vi "Scan1.vi"() -> ()   [LabVIEW 2022 SP3]
uses:
  <vilib>/userdefined/High Color/IMAQdx.ctl
  <vilib>/Utility/file.llb/Write To Spreadsheet File (DBL).vi
  <vilib>/vision/driver/NI_Vision_Acquisition_Software.lvlib
  <resource>/objmgr/IMAQImage.rc
panel:
  in  "ExitSendCmd":bool
  out "Current File":path
  in  "Root File Name":string="Sample"
  in  "Display as wavelngth?":bool=TRUE
  in  "ActiveFlyCapControl":refnum<k7>(container)
  out "X axis":dbl[](array[numeric])
  in  "Tab Control":enum32{"Scan", "Motors"}(tab)
  in  "Save Option":bool=TRUE
  out "Remaining Minutes":i32
  out "Progress Bar":dbl(slide) scale=0.0..1.0
  in  "Sample #":u16
  out "Cross Plane Length (mm)":sgl=128.0 format="%.3f"
  out "Scan Plane Length (mm)":sgl=128.0 format="%.3f"
  in  "Distance between\nscan lines (mm)":sgl=1.0 min=0.06 max=1000 step=0.06
  in  "Distance between\nplanes (mm)":sgl=1.0 min=0.06 max=1000 step=0.06
  in  "number of planes":u16=1660
  in  "lines per plane":u16=1660 min=1
  out "current plane":u16
  out "current line":u16
  in  "Abort":bool
  in  "start scan":bool
  out "Image":T1(plugin-control)
  out "Spectra":cluster{"X":dbl[], "Spectral Amplitude":dbl[]}(graph)
  in  "Save Folder":path=path "D:/Scan Test"
  in  "Average#":i32=1 min=1
  in  "Exposure (*2.375 ms)":u16=2 format="%.3f"
  in  "Plane Axis":refnum<k7>(container)
  in  "Line axis":refnum<k7>(container)
  in  "Home Seq":bool
  in  "Go Home":bool
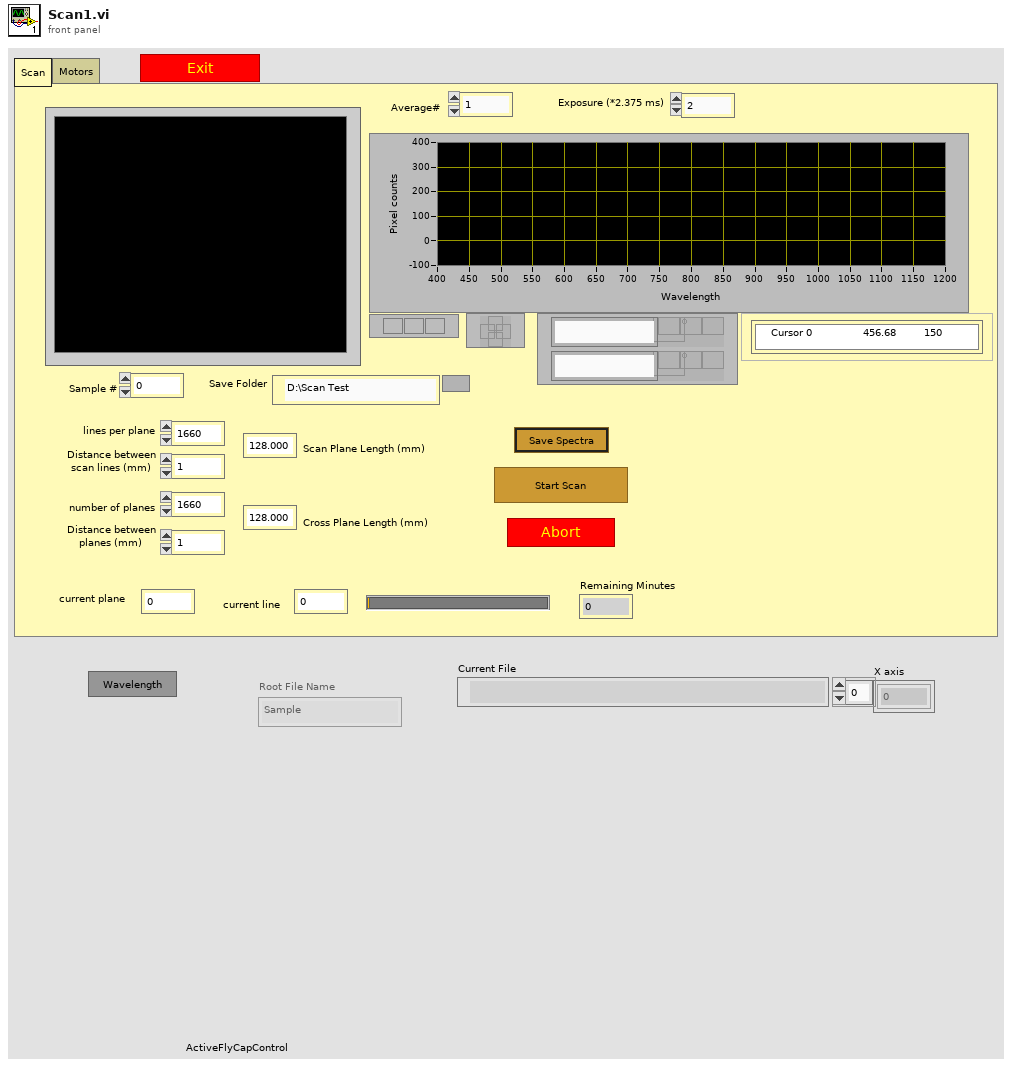
[diagram p1: front panel]
types:
  T1 = typedef "IMAQ Image.ctl" = refnum<image>
  T2 = typedef "IMAQdx.ctl" = refnum<k21>
  T3 = typedef "Image Type" = u32
  T4 = cluster{"X axis":dbl[], "Spectral Amplitude":dbl[]}
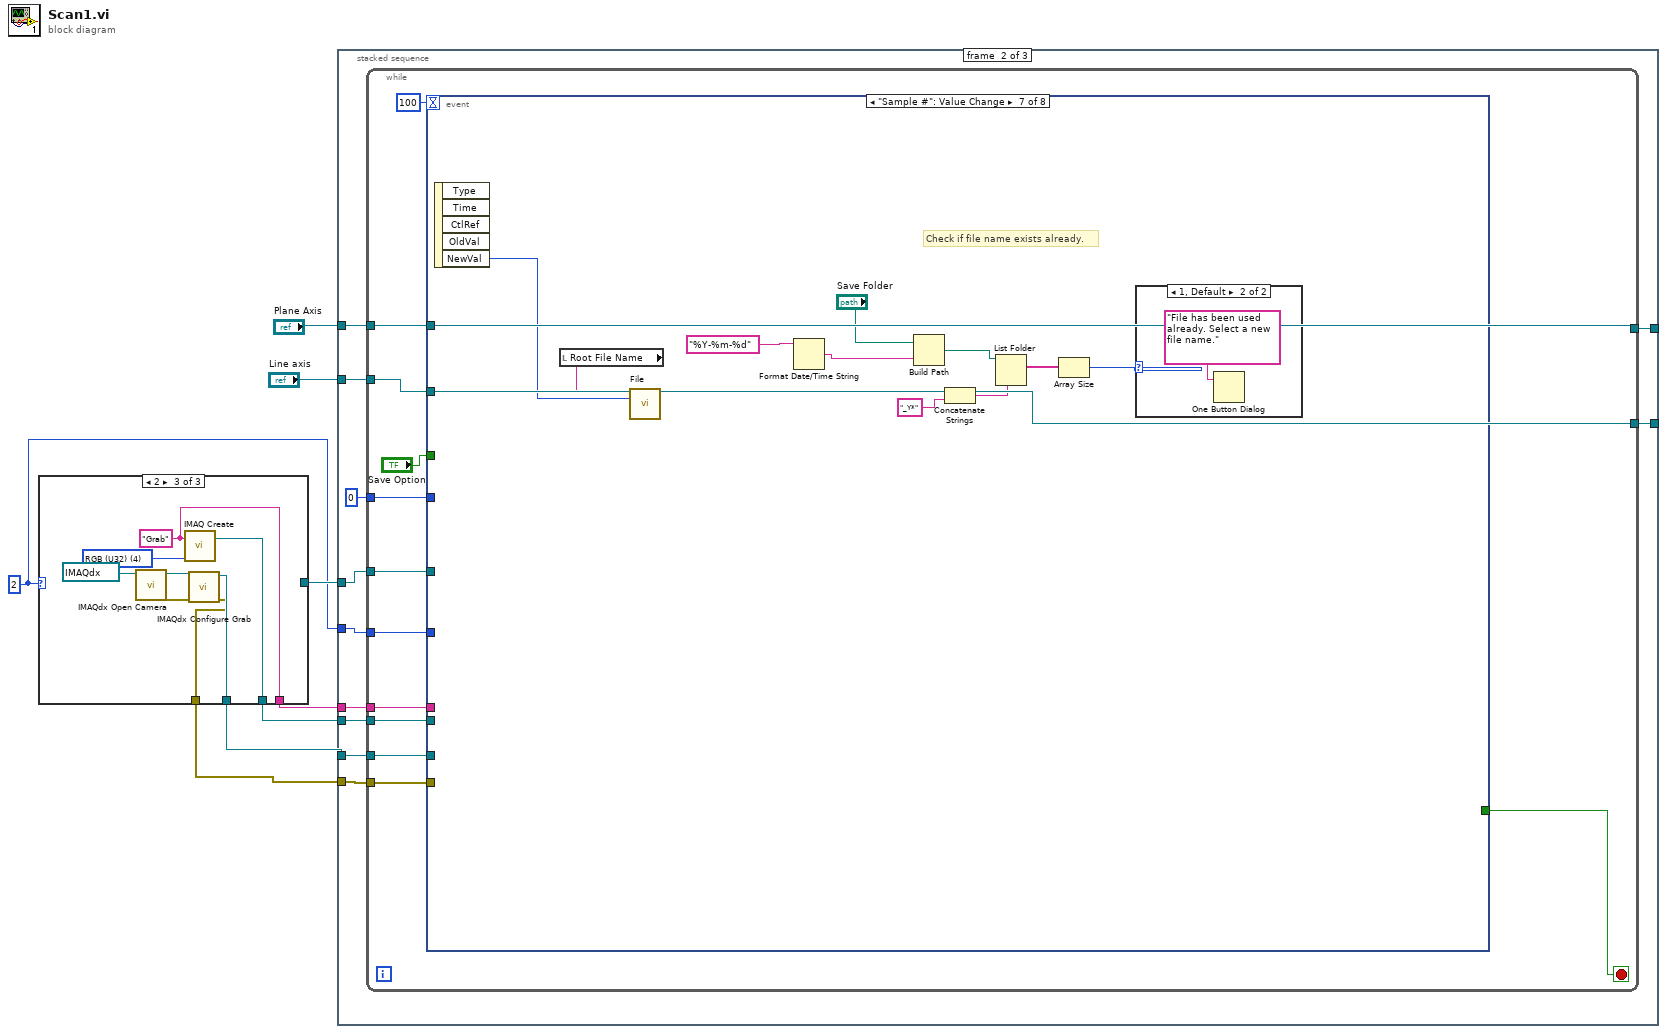
[diagram p0: block diagram]
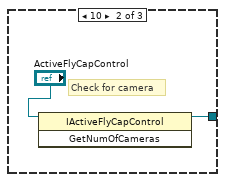
[diagram p3: hidden frame]
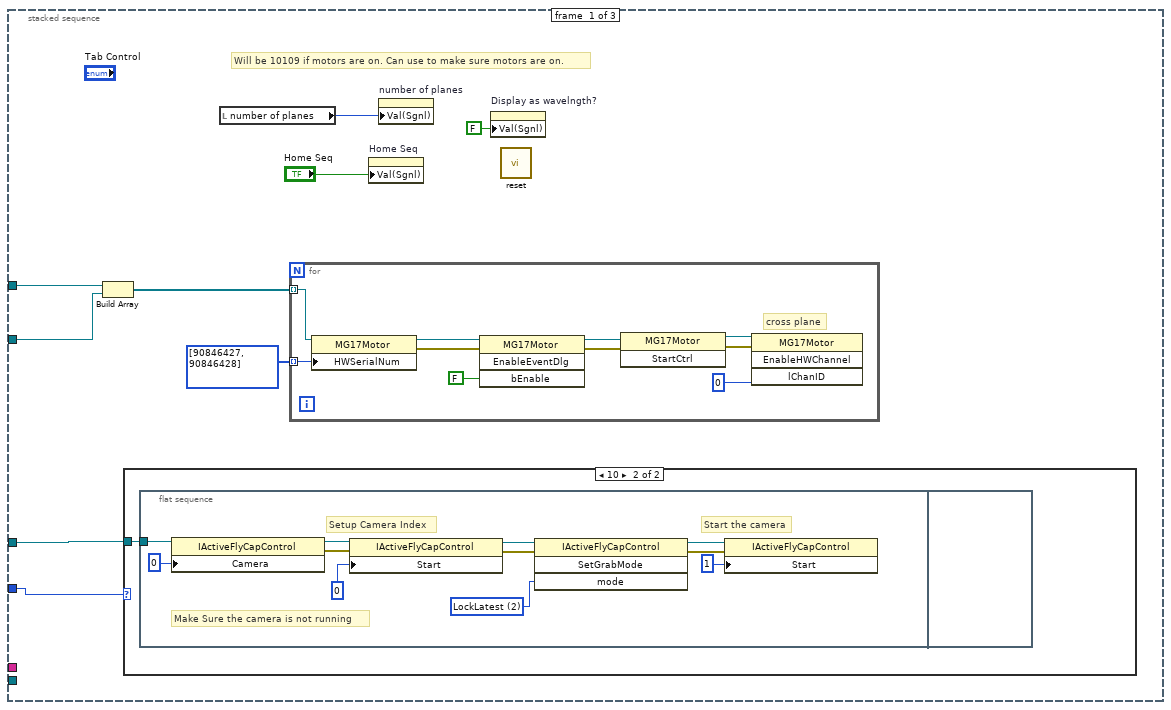
[diagram p4: hidden frame]
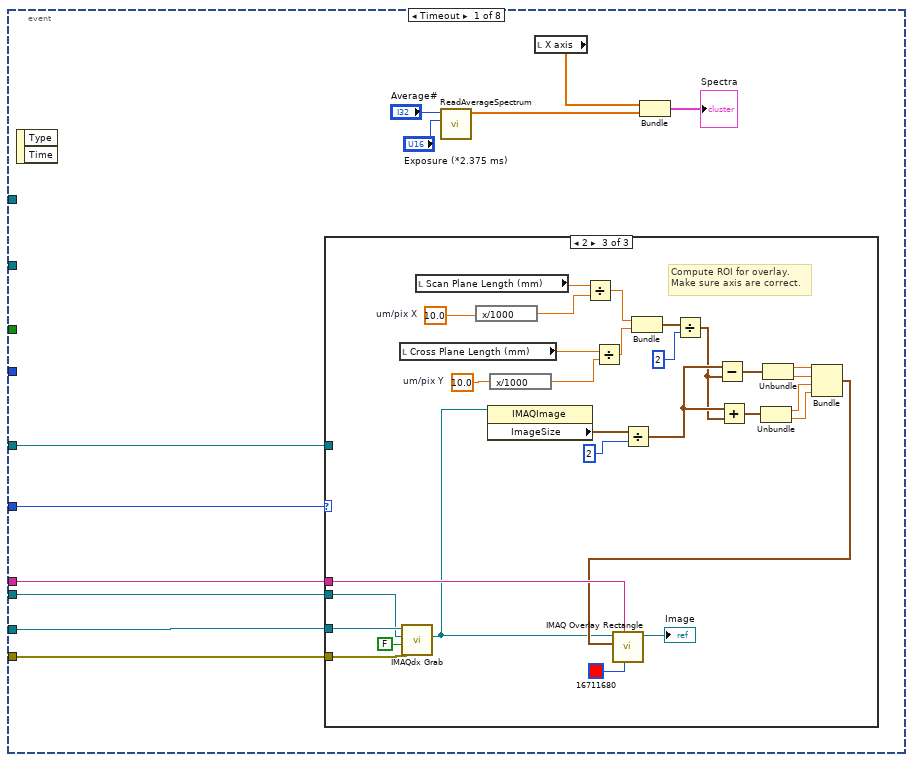
[diagram p6: hidden frame]
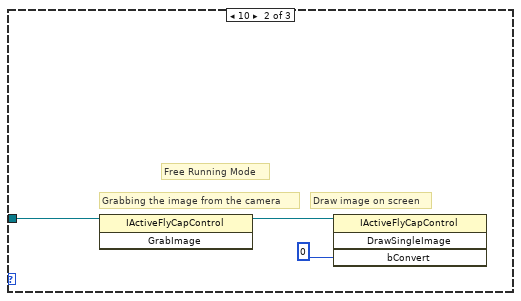
[diagram p8: hidden frame]
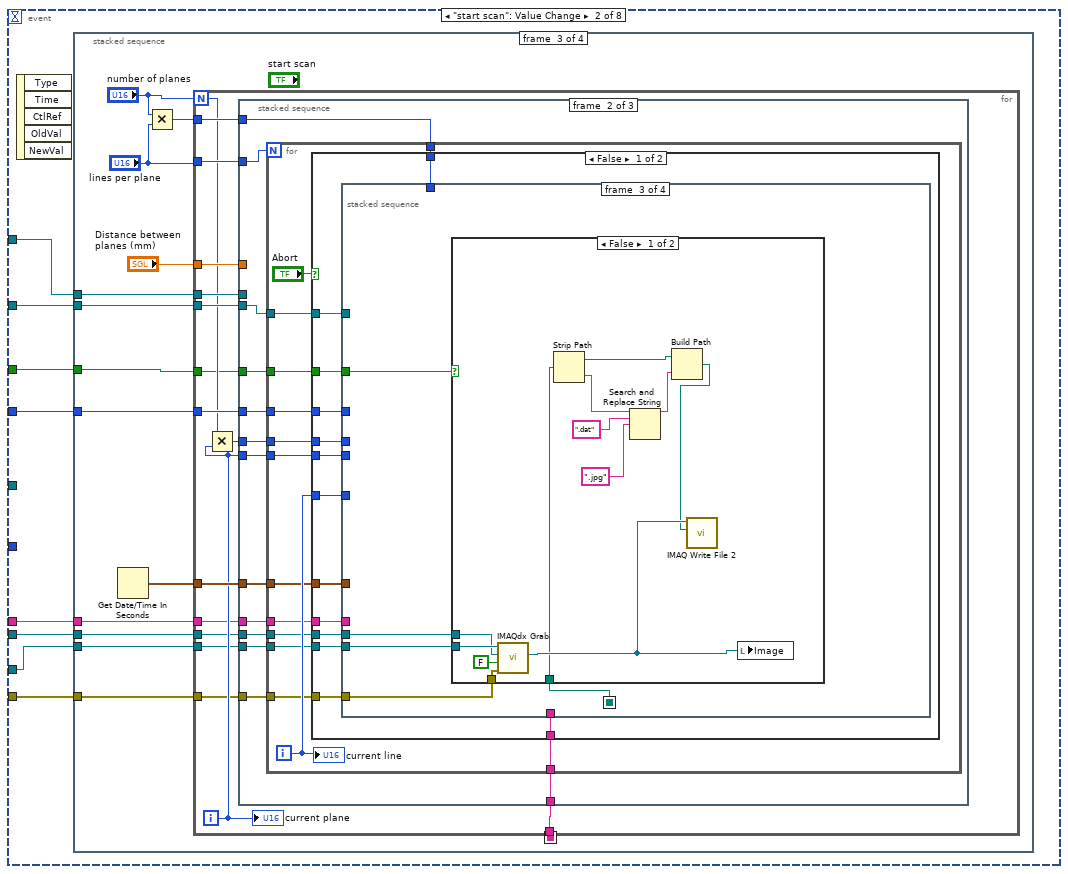
[diagram p9: hidden frame]
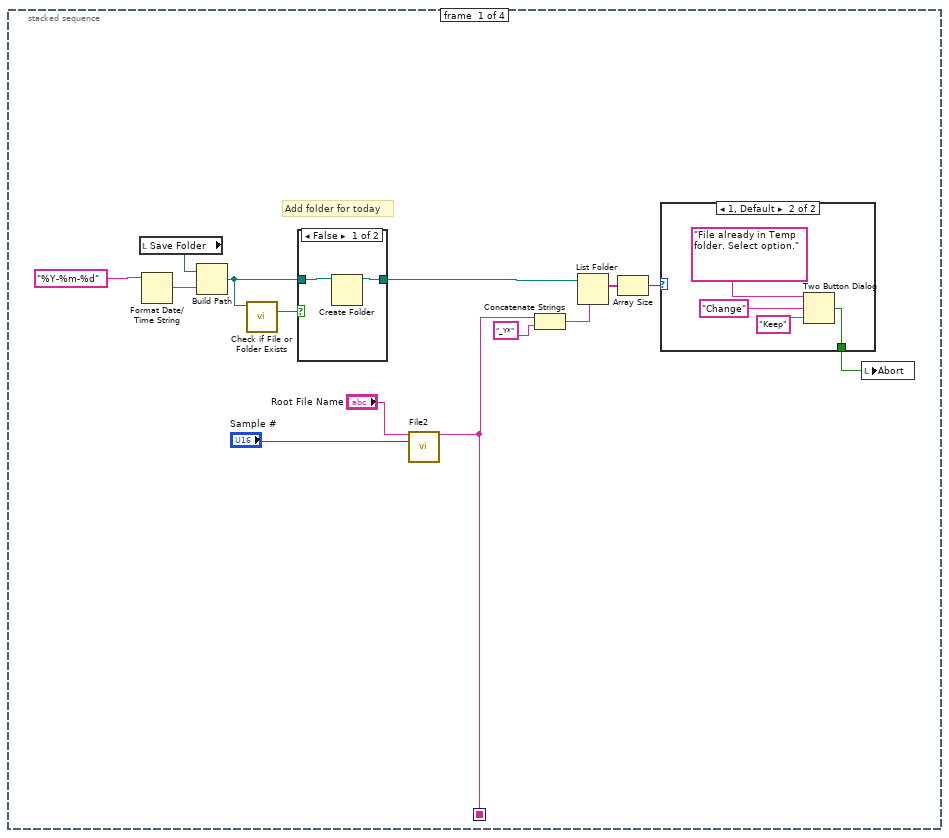
[diagram p10: hidden frame]
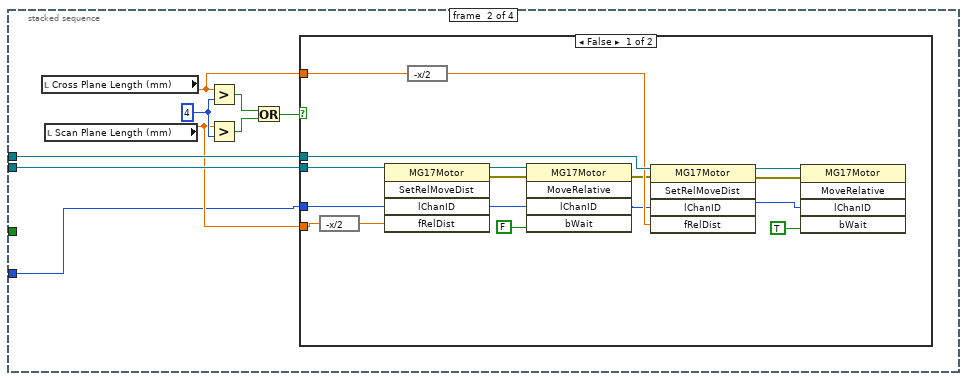
[diagram p13: hidden frame]
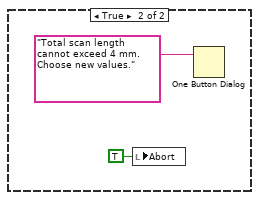
[diagram p14: hidden frame]
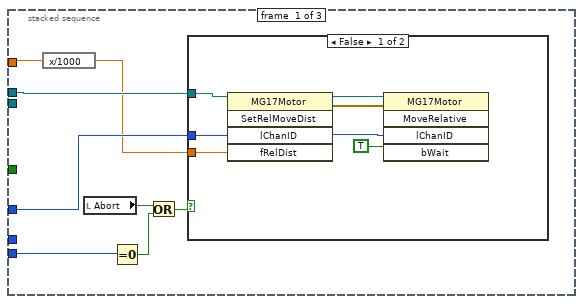
[diagram p15: hidden frame]
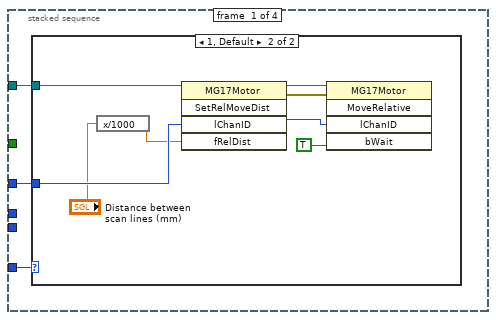
[diagram p17: hidden frame]
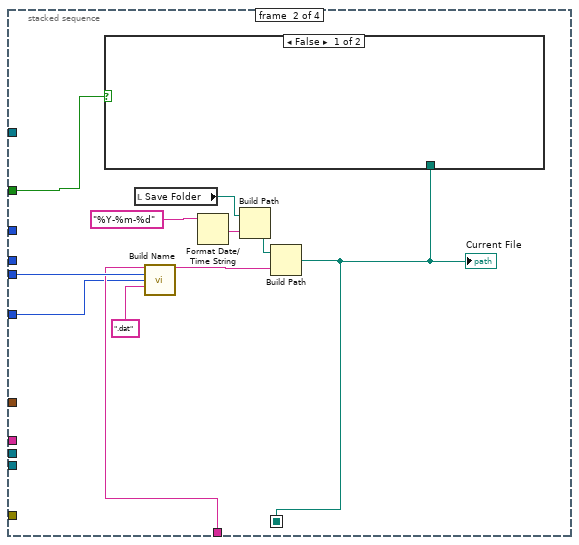
[diagram p19: hidden frame]
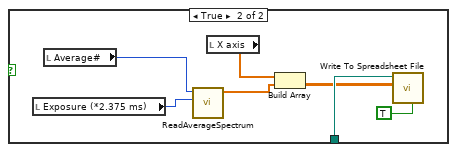
[diagram p20: hidden frame]
diagram:
  w1 = 2 ("bConvert")
  n1 = case shown="2" w1 {
    tunnel: [_ w10 _] -> w6
    tunnel: [_ _ w14] -> w5
    tunnel: [_ _ w13] -> w4
    tunnel: [_ _ w12] -> w3
    tunnel: [_ _ w11] -> w2
    frame 0, Default {
    }
    frame 10 {
      # "Check for camera"
      n2 = invoke class="IActiveFlyCapControl" method="GetNumOfCameras"(reference="ActiveFlyCapControl") -> (reference out=w10:refnum<k7>)  [unwired: 2 in, 2 out]
    }
    frame 2 {
      w15 = T3 4 items=["Grayscale (U8)", "Grayscale (I16)", "Grayscale (SGL)", "Complex (CSG)", "RGB (U32)", "HSL (U32)", "RGB (U64)", "Grayscale (U16)"] ("Image Type")
      w14 = "Grab" ("Image Name")
      n3 = call <vilib>:"IMAQdx Open Camera.vi"("Session In"=T2 "cam1") -> ("error out"=w17:errorcluster, "Session Out"=w18:T2)  [unwired: 2 in, 7 out]
      n4 = call "IMAQ Create"("Image Name"=w14, "Image Type"=w15) -> ("New Image"=w13:T1)  [unwired: 2 in, 2 out]
      n5 = call <vilib>:"IMAQdx Configure Grab.vi"("error in"=w17, "Session In"=w18) -> ("error out"=w11:errorcluster, "Session Out"=w12:T2)  [unwired: 1 in, 7 out]
    }
  }
  n6 = stacked-sequence {
    tunnel: [_ w59 _] -> _
    tunnel: [_ w58 _] -> _
    tunnel: w6 -> [w22 w57 w432]
    tunnel: "Plane Axis" -> [w20 w56 w431]
    tunnel: "Line axis" -> [w21 w55 w430]
    tunnel: w3 -> [_ w54 w428]
    tunnel: w4 -> [_ w53 w429]
    tunnel: w2 -> [_ w51 w427]
    tunnel: w5 -> [_ w52 _]
    tunnel: w1 -> [w19 w50 w426]
    frame #0 {
      # "Will be 10109 if motors are on. Can use to make sure motors are on."
      n7 = Build Array(w20, w21) -> (w23:refnum<k7>[])
      n8 = case shown="10" w19 {
        tunnel: w22 -> [_ w28]
        frame 0, Default {
        }
        frame 10 {
          n9 = flat-sequence {
            tunnel: w28 -> [w29]
            frame #0 {
              w32 = 2 items=["FreeRunning", "LockNext", "LockLatest"] ("mode")
              # "Make Sure the camera is not running"
              # "Setup Camera Index"
              # "Start the camera"
              n10 = property class="IActiveFlyCapControl"(reference=w29, "Camera"=0 ("Start")) -> (reference out=w35:refnum<k7>, error out=w37:errorcluster)  [unwired: 1 in]
              n11 = property class="IActiveFlyCapControl"(reference=w35, error in=w37, "Start"=0 ("Camera")) -> (reference out=w33:refnum<k7>, error out=w34:errorcluster)
              n12 = invoke class="IActiveFlyCapControl" method="SetGrabMode"(reference=w33, error in=w34, "mode"=w32) -> (reference out=w36:refnum<k7>, error out=w38:errorcluster)  [unwired: 1 in, 2 out]
              n13 = property class="IActiveFlyCapControl"(reference=w36, error in=w38, "Start"=1) -> ()  [unwired: 2 out]
            }
            frame #1 {
            }
          }
        }
      }
      n14 = local read "number of planes"() -> (w26:u16)
      n15 = for {
        tunnel: i32[] [90846427, 90846428] -> [w41] mode=indexing
        tunnel: w23 -> [w42] mode=indexing
        # "cross plane"
        n16 = property class="MG17Motor"(reference=w42, "HWSerialNum"=w41) -> (reference out=w40:refnum<k7>, error out=w45:errorcluster)  [unwired: 1 in]
        n17 = invoke class="MG17Motor" method="EnableEventDlg"(reference=w40, error in=w45, "bEnable"=FALSE ("pbCommsOK")) -> (reference out=w44:refnum<k7>, error out=w43:errorcluster)  [unwired: 1 in, 2 out]
        n18 = invoke class="MG17Motor" method="StartCtrl"(reference=w44, error in=w43) -> (reference out=w49:refnum<k7>, error out=w48:errorcluster)  [unwired: 1 in, 1 out]
        n19 = invoke class="MG17Motor" method="EnableHWChannel"(reference=w49, error in=w48, "lChanID"=0) -> ()  [unwired: 1 in, 4 out]
      }
      n20 = property on="Home Seq" class="Bool (strict)"("Val(Sgnl)"="Home Seq") -> ()  [unwired: 2 in, 2 out]
      n21 = property on="number of planes" class="DigNum (strict)"("Val(Sgnl)"=w26) -> ()  [unwired: 2 in, 2 out]
      n22 = property on="Display as wavelngth?" class="Bool (strict)"("Val(Sgnl)"=FALSE ("Value (Signaling)")) -> ()  [unwired: 2 in, 2 out]
      n23 = call "reset.vi"() -> ()  [unwired: 1 in]
    }
    frame #1 {
      n24 = while {
        tunnel: w55 -> [w69]
        tunnel: w56 -> [w70]
        tunnel: 0 ("lChanID") -> [w71]
        tunnel: [w69] -> w59
        tunnel: [w70] -> w58
        tunnel: w57 -> [w67]
        tunnel: w54 -> [w65]
        tunnel: w53 -> [w66]
        tunnel: w52 -> [w64]
        tunnel: w51 -> [w63]
        tunnel: w50 -> [w62]
        stop <- w72 stop-if-true
        n25 = event shown="[6] \"Sample #\": Value Change" {
          selector: _ -> [_ _ _ _ _ _ _ _]
          dyn-events: _ -> [_ _ _ _ _ _ _ _]
          timeout: 100 -> [_ _ _ _ _ _ _ _]
          tunnel: w69 -> [_ w121 w338 _ w371 _ _ _]
          tunnel: w70 -> [_ w123 w337 _ w372 _ _ _]
          tunnel: [_ _ _ "ExitSendCmd" _ _ _ _] -> w72
          tunnel: w71 -> [_ w122 w333 _ w368 _ _ _]
          tunnel: w67 -> [w83 _ _ _ _ _ _ _]
          tunnel: w66 -> [w76 w118 _ _ _ _ _ _]
          tunnel: w65 -> [w77 w120 _ _ _ _ _ _]
          tunnel: w64 -> [w75 w117 _ _ _ _ _ _]
          tunnel: w63 -> [w74 w119 _ _ _ _ _ _]
          tunnel: w62 -> [w73 _ _ _ _ _ _ _]
          tunnel: "Save Option" -> [_ w116 _ _ _ _ _ _]
          event Timeout {
            n26 = event-data() -> ()  [unwired: 1 in, 2 out]
            n27 = case shown="2" w73 {
              tunnel: w83 -> [_ w85 _]
              tunnel: w77 -> [_ _ w112]
              tunnel: w76 -> [_ _ w109]
              tunnel: w75 -> [_ _ w114]
              tunnel: w74 -> [_ _ w110]
              frame 0, Default {
              }
              frame 10 {
                # "Draw image on screen"
                # "Grabbing the image from the camera"
                # "Free Running Mode"
                n28 = invoke class="IActiveFlyCapControl" method="GrabImage"(reference=w85) -> (reference out=w84:refnum<k7>)  [unwired: 2 in, 2 out]
                n29 = invoke class="IActiveFlyCapControl" method="DrawSingleImage"(reference=w84, "bConvert"=0) -> ()  [unwired: 2 in, 4 out]
              }
              frame 2 {
                w104 = 10.0  # um/pix Y
                w105 = 10.0  # um/pix X
                # "Compute ROI for overlay.\nMake sure axis are correct."
                n30 = local read "Cross Plane Length (mm)"() -> (w88:sgl)
                n31 = call <vilib>:"IMAQdx Grab.vi"("error in"=w110, "Wait for Next Buffer? (Yes)"=FALSE, "Image In"=w109, "Session In"=w112) -> ("Image Out"=w89:T1)  [unwired: 7 out]
                n32 = local read "Scan Plane Length (mm)"() -> (w106:sgl)
                n33 = expression code="x/1000"(w105) -> (w103:dbl)
                n34 = property class="IMAQImage"(reference=w89) -> ("ImageSize"=w108:cluster{"x":i32, "y":i32})  [unwired: 1 in, 2 out]
                n35 = expression code="x/1000"(w104) -> (w87:dbl)
                n36 = Divide(x=w106, y=w103) -> (x/y=w102:dbl)
                n37 = Divide(x=w88, y=w87) -> (x/y=w101:dbl)
                n38 = Divide(x=w108, y=2) -> (x/y=w98:cluster{"x":dbl, "y":dbl})
                n39 = Bundle(w102, w101) -> (w100:cluster{dbl, dbl})  [unwired: 1 in]
                n40 = Divide(x=w100, y=2) -> (x/y=w97:cluster{dbl, dbl})
                n41 = Subtract(x=w98, y=w97) -> (x-y=w96:cluster{dbl, dbl})
                n42 = Add(x=w98, y=w97) -> (x+y=w95:cluster{dbl, dbl})
                n43 = Unbundle(w95) -> (w92:dbl, w91:dbl)
                n44 = Unbundle(w96) -> (w94:dbl, w93:dbl)
                n45 = Bundle(w94, w93, w92, w91) -> (w90:cluster{dbl, dbl, dbl, dbl})  [unwired: 1 in]
                n46 = call "IMAQ Overlay Rectangle"("Color"=u32 16711680, "Group"=w114, "Rectangle"=w90, "Image"=w89) -> ("Image Out"=→"Image":T1)  [unwired: 6 in, 1 out]
              }
            }
            n47 = call "ReadAverageSpectrum.vi"("Exposure (*2.375 ms)"="Exposure (*2.375 ms)", "Average#"="Average#") -> ("Spectral Amplitude"=w78:dbl[])  [unwired: 9 in]
            n48 = local read "X axis"() -> (w82:dbl[])
            n49 = Bundle("X axis"=w82, "Spectral Amplitude"=w78) -> (→"Spectra":T4)  [unwired: 1 in]
          }
          event "start scan": Value Change {
            n50 = event-data() -> ()  [unwired: 1 in, 5 out]
            n51 = stacked-sequence {
              seq-local: [w129 _ _ _] -> [_ _ w182 _]
              tunnel: w123 -> [_ w149 w186 _]
              tunnel: w121 -> [_ w150 w184 _]
              tunnel: w122 -> [_ w145 w183 _]
              tunnel: w120 -> [_ _ w177 _]
              tunnel: w119 -> [_ _ w176 _]
              tunnel: w118 -> [_ _ w175 _]
              tunnel: w117 -> [_ _ w174 _]
              tunnel: w116 -> [_ _ w173 _]
              frame #0 {
                # "Add folder for today"
                n52 = local read "Save Folder"() -> (w131:path)
                n53 = Format Date/Time String(time format string (%c)="%Y-%m-%d") -> (date/time string=w132:string)  [unwired: 2 in]
                n54 = Build Path(base path=w131, name or relative path=w132) -> (appended path=w126:path)
                n55 = call <vilib>:"Check if File or Folder Exists.vi"("path"=w126) -> ("file or folder exists?"=w125:bool)  [unwired: 8 in, 2 out]
                n56 = case shown="False" w125 {
                  tunnel: w126 -> [w143 w144]
                  tunnel: [w142 w144] -> w130
                  frame False {
                    n57 = Create Folder(path (use dialog)=w143) -> (created path=w142:path)  [unwired: 2 in, 2 out]
                  }
                  frame True {
                  }
                }
                n58 = call "File2"("Beginning Text"="Root File Name", "d"="Sample #") -> ("Result"=w129:string)  [unwired: 12 in, 1 out]
                n59 = Concatenate Strings(w129, "_Y*") -> (w137:string)
                n60 = List Folder(path=w130, pattern=w137) -> (filenames=w136:string[])  [unwired: 1 in, 4 out]
                n61 = Array Size(array=w136) -> (size(s)=w135:i32)
                n62 = case shown="1, Default" w135 {
                  tunnel: [_ w138] -> w133
                  frame 0 {
                  }
                  frame 1, Default {
                    n63 = Two Button Dialog(message="File already in Temp folder. Select option.", 1:"Keep" ("F button name (\"Cancel\")"), 2:"Change" ("T button name (\"OK\")")) -> (T button?=w138:bool)
                  }
                }
                n64 = local write "Abort"(w133) -> ()
              }
              frame #1 {
                w152 = 4
                n65 = local read "Cross Plane Length (mm)"() -> (w148:sgl)
                n66 = local read "Scan Plane Length (mm)"() -> (w147:sgl)
                n67 = Greater?(x=w148, y=w152) -> (0:w153:bool)
                n68 = Greater?(x=w147, y=w152) -> (0:w151:bool)
                n69 = Or(x=w153, y=w151) -> (x .or. y?=w146:bool)
                n70 = case shown="False" w146 {
                  tunnel: w150 -> [w164 _]
                  tunnel: w149 -> [w163 _]
                  tunnel: w145 -> [w158 _]
                  tunnel: w148 -> [w162 _]
                  tunnel: w147 -> [w161 _]
                  frame False {
                    n71 = expression code="-x/2"(w161) -> (w160:sgl)
                    n72 = invoke class="MG17Motor" method="SetRelMoveDist"(reference=w164, "lChanID"=w158, "fRelDist"=w160) -> (reference out=w169:refnum<k7>, error out=w155:errorcluster, "lChanID"=w168:i32)  [unwired: 2 in, 2 out]
                    n73 = expression code="-x/2"(w162) -> (w159:sgl)
                    n74 = invoke class="MG17Motor" method="MoveRelative"(reference=w169, error in=w155, "lChanID"=w168, "bWait"=FALSE) -> (error out=w156:errorcluster, "lChanID"=w154:i32)  [unwired: 1 in, 3 out]
                    n75 = invoke class="MG17Motor" method="SetRelMoveDist"(reference=w163, error in=w156, "lChanID"=w154, "fRelDist"=w159) -> (reference out=w166:refnum<k7>, error out=w157:errorcluster, "lChanID"=w165:i32)  [unwired: 1 in, 2 out]
                    n76 = invoke class="MG17Motor" method="MoveRelative"(reference=w166, error in=w157, "lChanID"=w165, "bWait"=TRUE) -> ()  [unwired: 1 in, 5 out]
                  }
                  frame True {
                    n77 = local write "Abort"(TRUE ("Abort")) -> ()
                    n78 = One Button Dialog(message="Total scan length cannot exceed 4 mm. Choose new values.") -> ()  [unwired: 1 in, 1 out]
                  }
                }
              }
              frame #2 {
                n79 = Get Date/Time In Seconds() -> (seconds since 1Jan1904=w178:timestamp)
                n80 = Multiply(x="number of planes", y="lines per plane") -> (x*y=w179:u16)
                n81 = for {
                  N: "number of planes" -> [w194]
                  tunnel: "lines per plane" -> [w202]
                  tunnel: w186 -> [w201]
                  tunnel: "Distance between\nplanes (mm)" -> [w200]
                  tunnel: w184 -> [w199]
                  tunnel: w183 -> [w198]
                  tunnel: w182 -> [w197]
                  tunnel: w179 -> [w196]
                  tunnel: w178 -> [w195]
                  tunnel: w177 -> [w191]
                  tunnel: w176 -> [w190]
                  tunnel: w175 -> [w189]
                  tunnel: w174 -> [w188]
                  tunnel: w173 -> [w187]
                  i -> [w193]
                  n82 = Multiply(x=w194, y=w193) -> (x*y=w192:i32)
                  n83 = stacked-sequence {
                    tunnel: w202 -> [_ w230 _]
                    tunnel: w201 -> [w210 _ _]
                    tunnel: w200 -> [w208 _ _]
                    tunnel: w199 -> [_ w229 w317]
                    tunnel: w198 -> [w209 w228 w318]
                    tunnel: w193 -> [w203 w227 _]
                    tunnel: w197 -> [_ w226 _]
                    tunnel: w196 -> [_ w225 _]
                    tunnel: w195 -> [_ w224 _]
                    tunnel: w192 -> [_ w223 _]
                    tunnel: w191 -> [_ w222 _]
                    tunnel: w190 -> [_ w221 _]
                    tunnel: w189 -> [_ w220 _]
                    tunnel: w188 -> [_ w219 _]
                    tunnel: w187 -> [_ w218 _]
                    frame #0 {
                      n84 = expression code="x/1000"(w208) -> (w207:sgl)
                      n85 = local read "Abort"() -> (w206:bool)
                      n86 = Equal To 0?(x=w203) -> (x = 0?=w205:bool)
                      n87 = Or(x=w206, y=w205) -> (x .or. y?=w204:bool)
                      n88 = case shown="False" w204 {
                        tunnel: w210 -> [w216 _]
                        tunnel: w209 -> [w213 _]
                        tunnel: w207 -> [w212 _]
                        frame False {
                          n89 = invoke class="MG17Motor" method="SetRelMoveDist"(reference=w216, "lChanID"=w213, "fRelDist"=w212) -> (reference out=w215:refnum<k7>, error out=w211:errorcluster, "lChanID"=w214:i32)  [unwired: 2 in, 2 out]
                          n90 = invoke class="MG17Motor" method="MoveRelative"(reference=w215, error in=w211, "lChanID"=w214, "bWait"=TRUE) -> ()  [unwired: 1 in, 5 out]
                        }
                        frame True {
                        }
                      }
                    }
                    frame #1 {
                      n91 = for {
                        N: w230 -> [_]
                        tunnel: w229 -> [w244]
                        tunnel: w228 -> [w243]
                        tunnel: w227 -> [w240]
                        tunnel: w226 -> [w239]
                        tunnel: w225 -> [w238]
                        tunnel: w224 -> [w237]
                        tunnel: w223 -> [w236]
                        tunnel: w222 -> [w235]
                        tunnel: w221 -> [w234]
                        tunnel: w220 -> [w233]
                        tunnel: w219 -> [w232]
                        tunnel: w218 -> [w231]
                        i -> [w241]
                        n92 = case shown="False" "Abort" {
                          tunnel: w244 -> [w257 _]
                          tunnel: w243 -> [w256 _]
                          tunnel: w241 -> [w255 _]
                          tunnel: w240 -> [w254 _]
                          tunnel: w239 -> [w253 _]
                          tunnel: w238 -> [w252 _]
                          tunnel: w237 -> [w251 _]
                          tunnel: w236 -> [w250 _]
                          tunnel: w235 -> [w249 _]
                          tunnel: w234 -> [w248 _]
                          tunnel: w233 -> [w247 _]
                          tunnel: w232 -> [w246 _]
                          tunnel: w231 -> [w245 _]
                          frame False {
                            n93 = stacked-sequence {
                              seq-local: [_ w276 _ _] -> [_ _ w288 _]
                              tunnel: w257 -> [w260 _ _ _]
                              tunnel: w256 -> [w259 _ _ _]
                              tunnel: w255 -> [w258 w277 _ w314]
                              tunnel: w254 -> [_ w279 _ _]
                              tunnel: w253 -> [_ w278 _ _]
                              tunnel: w252 -> [_ _ _ w315]
                              tunnel: w251 -> [_ _ _ w311]
                              tunnel: w250 -> [_ _ _ w312]
                              tunnel: w249 -> [_ _ w291 _]
                              tunnel: w248 -> [_ _ w290 _]
                              tunnel: w247 -> [_ _ w289 _]
                              tunnel: w246 -> [_ _ _ _]
                              tunnel: w245 -> [_ w269 w287 _]
                              frame #0 {
                                n94 = case shown="1, Default" w258 {
                                tunnel: w260 -> [_ w265]
                                tunnel: w259 -> [_ w264]
                                frame 0 {
                                }
                                frame 1, Default {
                                n95 = expression code="x/1000"("Distance between\nscan lines (mm)") -> (w262:sgl)
                                n96 = invoke class="MG17Motor" method="SetRelMoveDist"(reference=w265, "lChanID"=w264, "fRelDist"=w262) -> (reference out=w267:refnum<k7>, error out=w263:errorcluster, "lChanID"=w266:i32)  [unwired: 2 in, 2 out]
                                n97 = invoke class="MG17Motor" method="MoveRelative"(reference=w267, error in=w263, "lChanID"=w266, "bWait"=TRUE) -> ()  [unwired: 1 in, 5 out]
                                }
                                }
                              }
                              frame #1 {
                                n98 = local read "Save Folder"() -> (w271:path)
                                n99 = call "Build Name"("Beginning Text"=w278, "plane"=w279, "line"=w277, "file_EXT"=".dat") -> ("Result"=w274:string)  [unwired: 10 in, 1 out]
                                n100 = Format Date/Time String(time format string (%c)="%Y-%m-%d") -> (date/time string=w273:string)  [unwired: 2 in]
                                n101 = Build Path(base path=w271, name or relative path=w273) -> (appended path=w270:path)
                                n102 = Build Path(base path=w270, name or relative path=w274) -> (appended path=w276:path)
                                "Current File" <- w276
                                n103 = case shown="False" w269 {
                                tunnel: w276 -> [_ w286]
                                frame False {
                                }
                                frame True {
                                n104 = local read "Exposure (*2.375 ms)"() -> (w280:u16)
                                n105 = local read "Average#"() -> (w281:i32)
                                n106 = call "ReadAverageSpectrum.vi"("Exposure (*2.375 ms)"=w280, "Average#"=w281) -> ("Spectral Amplitude"=w284:dbl[])  [unwired: 9 in]
                                n107 = local read "X axis"() -> (w285:dbl[])
                                n108 = Build Array(w285, w284) -> (w283:dbl[][])
                                n109 = call-poly <vilib>:"Write To Spreadsheet File.vi"("transpose? (no:F)"=TRUE, "2D data"=w283, "file path (dialog if empty)"=w286) -> ()  [unwired: 5 in, 1 out]
                                }
                                }
                              }
                              frame #2 {
                                n110 = case shown="False" w287 {
                                tunnel: w291 -> [w302 _]
                                tunnel: w290 -> [w301 _]
                                tunnel: w289 -> [w300 _]
                                tunnel: w288 -> [w298 _]
                                frame False {
                                n111 = call <vilib>:"IMAQdx Grab.vi"("error in"=w301, "Wait for Next Buffer? (Yes)"=FALSE, "Image In"=w300, "Session In"=w302) -> ("Image Out"=w299:T1)  [unwired: 7 out]
                                n112 = Strip Path(path=w298) -> (stripped path=w295:path, name=w297:string)
                                n113 = Search and Replace String(input string=w297, search string=".dat", replace string=".jpg" ("search string")) -> (result string=w294:string)  [unwired: 5 in, 3 out]
                                n114 = Build Path(base path=w295, name or relative path=w294) -> (appended path=w293:path)
                                n115 = call-poly "IMAQ Write File 2"("File Path"=w293, "Image"=w299) -> ()  [unwired: 8 in, 2 out]
                                n116 = local write "Image"(w299) -> ()
                                }
                                frame True {
                                }
                                }
                              }
                              frame #3 {
                                n117 = Get Date/Time In Seconds() -> (seconds since 1Jan1904=w310:timestamp)
                                n118 = Add(x=w312, y=w314) -> (x+y=w313:i32)
                                n119 = Subtract(x=w310, y=w311) -> (x-y=w309:dbl)
                                n120 = Divide(x=w313, y=w315) -> (x/y=w307:dbl)
                                "Progress Bar" <- w307
                                n121 = Divide(x=w309, y=60) -> (x/y=w305:dbl)
                                n122 = Divide(x=w305, y=w307) -> (x/y=w306:dbl)
                                n123 = Subtract(x=w306, y=w305) -> (x-y=→"Remaining Minutes":dbl)
                              }
                            }
                          }
                          frame True {
                          }
                        }
                        "current line" <- w241
                      }
                    }
                    frame #2 {
                      n124 = local read "Scan Plane Length (mm)"() -> (w319:sgl)
                      n125 = Negate(x=w319) -> (-x=w316:sgl)
                      n126 = invoke class="MG17Motor" method="SetRelMoveDist"(reference=w317, "lChanID"=w318, "fRelDist"=w316) -> (reference out=w321:refnum<k7>, error out=w323:errorcluster, "lChanID"=w322:i32)  [unwired: 2 in, 2 out]
                      n127 = invoke class="MG17Motor" method="MoveRelative"(reference=w321, error in=w323, "lChanID"=w322, "bWait"=TRUE) -> ()  [unwired: 1 in, 5 out]
                    }
                  }
                  "current plane" <- w193
                }
              }
              frame #3 {
                n128 = local read "Abort"() -> (w324:bool)
                n129 = case shown="False" w324 {
                  frame False {
                    n130 = local read "Sample #"() -> (w326:u16)
                    n131 = Increment(x=w326) -> (x+1=w327:u16)
                    n132 = local write "Sample #"(w327) -> ()
                  }
                  frame True {
                    n133 = local write "Abort"(FALSE ("Abort")) -> ()
                  }
                }
                n134 = property on="Go Home" class="Bool (strict)"("Val(Sgnl)"="Go Home") -> ()  [unwired: 2 in, 2 out]
              }
            }
          }
          event "Home Seq": Value Change {
            n135 = event-data() -> ()  [unwired: 1 in, 5 out]
            n136 = invoke class="MG17Motor" method="GetStatusBits_Bits"(reference=w337, "lChanID"=w333) -> ("GetStatusBits_Bits"=w336:i32)  [unwired: 2 in, 3 out]
            n137 = Number To Boolean Array(number=w336) -> (Boolean array=w335:bool[])
            n138 = Index Array(array=w335, index=10) -> (element=w331:bool)
            n139 = case shown="True" w331 {
              tunnel: [_ w340] -> w330
              frame False {
              }
              frame True {
                n140 = Two Button Dialog(message="Home Sequence Was Already Performed", 1:"Override" ("F button name (\"Cancel\")")) -> (T button?=w340:bool)  [unwired: 1 in]
              }
            }
            n141 = local write "Home Seq"(FALSE ("Home Seq")) -> ()
            n142 = case shown="False" w330 {
              tunnel: w338 -> [w344 w357]
              tunnel: w333 -> [w346 _]
              tunnel: w337 -> [w345 w358]
              frame False {
                n143 = Build Array(w345, w344) -> (w343:refnum<k7>[])
                n144 = for {
                  tunnel: w346 -> [w356]
                  tunnel: w343 -> [w355] mode=indexing
                  tunnel: bool[] [FALSE, TRUE] -> [w354] mode=indexing
                  w352 = sgl 0.5  # pfPitch
                  w349 = 1  # plDirSense
                  w353 = 1  # plUnits
                  n145 = invoke class="MG17Motor" method="MoveHome"(reference=w355, "lChanID"=w356, "bWait"=w354) -> (reference out=w347:refnum<k7>)  [unwired: 2 in, 4 out]
                  n146 = invoke class="MG17Motor" method="SetStageAxisInfo"(reference=w347, "lChanID"=0 ("lLimitMode"), "fMinPos"=sgl 0.0, "fMaxPos"=sgl 4.0, "lUnits"=w353, "fPitch"=w352, "lDirSense"=w349) -> ()  [unwired: 2 in, 9 out]
                }
              }
              frame True {
                n147 = Build Array(w358, w357) -> (w359:refnum<k7>[])
                n148 = for {
                  tunnel: w359 -> [w360] mode=indexing
                  w365 = sgl 0.5  # pfPitch
                  w362 = 1  # plDirSense
                  w366 = 1  # plUnits
                  n149 = invoke class="MG17Motor" method="SetStageAxisInfo"(reference=w360, "lChanID"=0 ("lLimitMode"), "fMinPos"=sgl 0.0, "fMaxPos"=sgl 4.0, "lUnits"=w366, "fPitch"=w365, "lDirSense"=w362) -> ()  [unwired: 2 in, 9 out]
                }
              }
            }
            n150 = property on="Go Home" class="Bool (strict)"("Val(Sgnl)"=FALSE ("Value (Signaling)")) -> ()  [unwired: 2 in, 2 out]
          }
          event "ExitSendCmd": Value Change {
            n151 = event-data() -> ()  [unwired: 1 in, 5 out]
          }
          event "Go Home": Value Change {
            n152 = event-data() -> ()  [unwired: 1 in, 5 out]
            n153 = Build Array(w372, w371) -> (w370:refnum<k7>[])
            n154 = for {
              tunnel: w370 -> [w375] mode=indexing
              tunnel: bool[] [FALSE, TRUE] -> [w376] mode=indexing
              tunnel: w368 -> [w374]
              n155 = invoke class="MG17Motor" method="SetAbsMovePos"(reference=w375, "lChanID"=w374, "fAbsPos"=sgl 2.0) -> (reference out=w379:refnum<k7>, error out=w377:errorcluster, "lChanID"=w378:i32)  [unwired: 2 in, 2 out]
              n156 = invoke class="MG17Motor" method="MoveAbsolute"(reference=w379, error in=w377, "lChanID"=w378, "bWait"=w376) -> ()  [unwired: 1 in, 5 out]
            }
            n157 = local write "Go Home"(FALSE ("Go Home")) -> ()
          }
          event "number of planes", "lines per plane", "Distance between\nscan lines (mm)", "Distance between\nplanes (mm)": Value Change {
            w382 = 4
            n158 = event-data() -> ()  [unwired: 1 in, 5 out]
            n159 = local read "Distance between\nscan lines (mm)"() -> (w393:sgl)
            n160 = local read "Distance between\nplanes (mm)"() -> (w394:sgl)
            n161 = local read "lines per plane"() -> (w387:u16)
            n162 = local read "number of planes"() -> (w388:u16)
            n163 = Decrement(x=w387) -> (x-1=w391:u16)
            n164 = Decrement(x=w388) -> (x-1=w392:u16)
            n165 = Multiply(x=w393, y=w391) -> (x*y=w389:sgl)
            n166 = Multiply(x=w394, y=w392) -> (x*y=w390:sgl)
            n167 = expression code="x/1000"(w390) -> (w386:sgl)
            "Cross Plane Length (mm)" <- w386
            n168 = expression code="x/1000"(w389) -> (w383:sgl)
            "Scan Plane Length (mm)" <- w383
            n169 = Greater?(x=w386, y=w382) -> (0:w385:bool)
            n170 = Greater?(x=w383, y=w382) -> (0:w381:bool)
            n171 = Or(x=w385, y=w381) -> (x .or. y?=w384:bool)
            n172 = case shown="True" w384 {
              frame False {
              }
              frame True {
                n173 = One Button Dialog(message="Total scan length cannot exceed 4 mm. Choose new values.") -> ()  [unwired: 1 in, 1 out]
              }
            }
          }
          event "Sample #": Value Change {
            # "Check if file name exists already."
            n174 = event-data() -> ("NewVal"=w397:u16)  [unwired: 1 in, 4 out]
            n175 = local read "Root File Name"() -> (w398:string)
            n176 = call "File"("Beginning Text"=w398, "d"=w397) -> ("Result"=w396:string)  [unwired: 12 in, 1 out]
            n177 = Format Date/Time String(time format string (%c)="%Y-%m-%d") -> (date/time string=w401:string)  [unwired: 2 in]
            n178 = Build Path(base path="Save Folder", name or relative path=w401) -> (appended path=w400:path)
            n179 = Concatenate Strings(w396, "_Y*") -> (w406:string)
            n180 = List Folder(path=w400, pattern=w406) -> (filenames=w405:string[])  [unwired: 1 in, 4 out]
            n181 = Array Size(array=w405) -> (size(s)=w399:i32)
            n182 = case shown="1, Default" w399 {
              frame 0 {
              }
              frame 1, Default {
                n183 = One Button Dialog(message="File has been used already. Select a new file name.") -> ()  [unwired: 1 in, 1 out]
              }
            }
          }
          event "Display as wavelngth?": Value Change {
            n184 = event-data() -> ()  [unwired: 1 in, 5 out]
            n185 = case shown="False" "Display as wavelngth?" {
              tunnel: u16 3712 -> [w412 w417]
              tunnel: [w411 w418] -> w409
              frame False {
                n186 = for {
                  N: w412 -> [_]
                  tunnel: [w413] -> w411 mode=indexing
                  i -> [w413]
                }
              }
              frame True {
                n187 = call "read_corr_coeff.vi"() -> ("A\n(Ax^2+Bx+C)"=w414:dbl, "B\n(Ax^2+Bx+C)"=w415:dbl, "C\n(Ax^2+Bx+C)"=w416:dbl)  [unwired: 1 in, 2 out]
                n188 = for {
                  N: w417 -> [_]
                  tunnel: w416 -> [w424]
                  tunnel: w415 -> [w423]
                  tunnel: w414 -> [w420]
                  tunnel: [w422] -> w418 mode=indexing
                  i -> [w421]
                  n189 = Multiply(x=w423, y=w421) -> (x*y=w425:dbl)
                  n190 = Compound Arithmetic op=MULTIPLY(w420, w421, w421) -> (w419:dbl)
                  n191 = Compound Arithmetic op=ADD(w424, w425, w419) -> (w422:dbl)
                }
              }
            }
            "X axis" <- w409
          }
        }
      }
    }
    frame #2 {
      n192 = case shown="2" w426 {
        tunnel: w432 -> [_ w434 _]
        tunnel: w429 -> [_ _ w438]
        tunnel: w428 -> [_ _ w437]
        tunnel: w427 -> [_ _ w436]
        frame 0, Default {
        }
        frame 10 {
          # "Stop the camera"
          n193 = property class="IActiveFlyCapControl"(reference=w434, "Start"=0) -> ()  [unwired: 1 in, 2 out]
        }
        frame 2 {
          n194 = call <vilib>:"IMAQdx Close Camera.vi"("error in"=w436, "Session In"=w437) -> ("error out"=w439:errorcluster)  [unwired: 9 out]
          n195 = call "Imaq Dispose"("Image"=w438, "error in (no error)"=w439) -> ()  [unwired: 4 in, 1 out]
        }
      }
      n196 = case shown="True" TRUE {
        tunnel: w431 -> [_ w441]
        tunnel: w430 -> [_ w440]
        frame False {
        }
        frame True {
          n197 = invoke class="MG17Motor" method="StopCtrl"(reference=w440) -> ()  [unwired: 2 in, 3 out]
          n198 = invoke class="MG17Motor" method="StopCtrl"(reference=w441) -> ()  [unwired: 2 in, 3 out]
        }
      }
    }
  }
